vi "4463 and 4464 sync test.vi"() -> ()   [LabVIEW 2015]
uses:
  <vilib>/Analysis/1siggen.llb/Ramp Pattern by Samples.vi
  <vilib>/DAQmx/write.llb/DAQmx Write (Analog 1D DBL 1Chan NSamp).vi
  <vilib>/DAQmx/read.llb/DAQmx Read (Analog 1D DBL 1Chan NSamp).vi
  <vilib>/DAQmx/create/channels.llb/DAQmx Create Channel (AI-Voltage-Basic).vi
  <vilib>/DAQmx/configure/timing.llb/DAQmx Timing (Sample Clock).vi
  <vilib>/DAQmx/create/channels.llb/DAQmx Create Channel (AO-Voltage-Basic).vi
  <vilib>/DAQmx/configure/trigger.llb/DAQmx Start Trigger (Digital Edge).vi
  <vilib>/DAQmx/miscellaneous.llb/DAQmx Fill In Error Info.vi
  <resource>/objmgr/daqmx.rc
  <vilib>/Analysis/NI_AALBase.lvlib
panel:
  out "Graph":dbl[](graph)
  in  "stop":bool
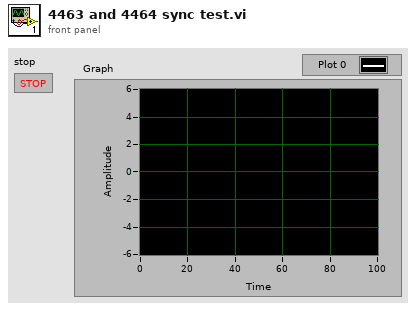
[diagram p1: front panel]
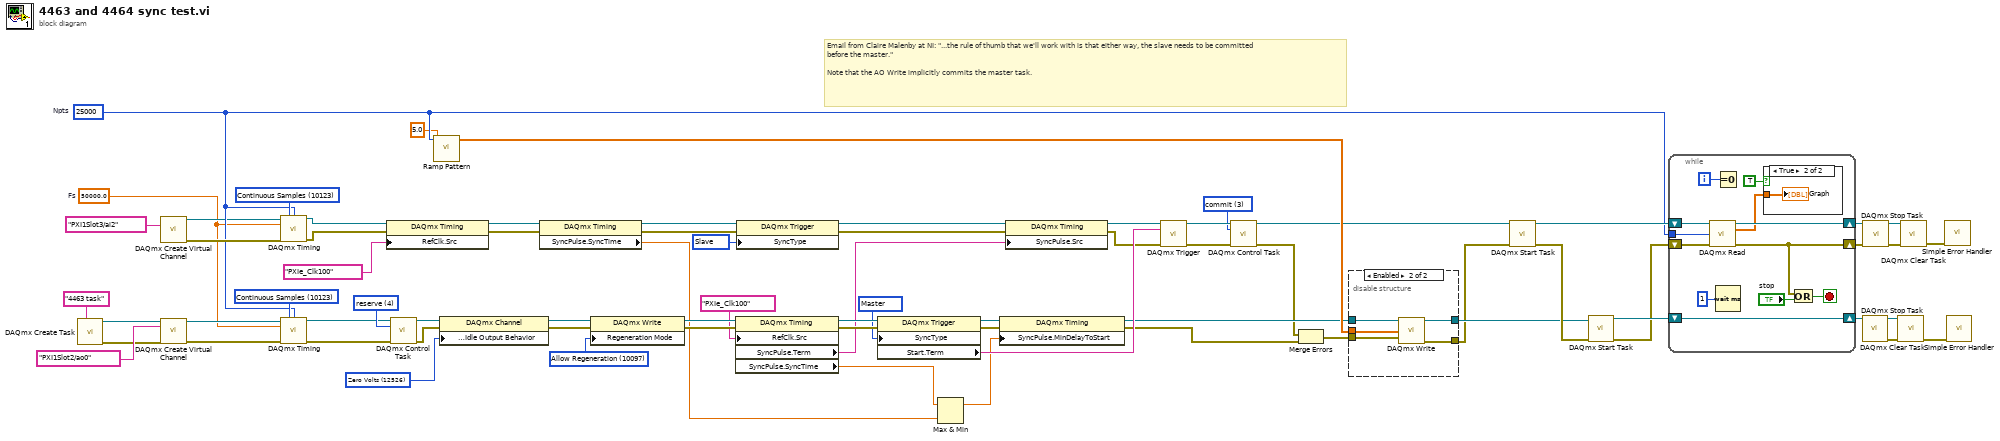
[diagram p0: block diagram]
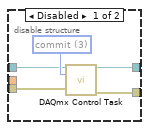
[diagram p2: hidden frame]
diagram:
  w1 = 3 items=["verify"=2, "reserve"=4, "commit"=3, "unreserve"=5, "abort"=6] ("action")
  w27 = 4 items=["verify"=2, "reserve"=4, "commit"=3, "unreserve"=5, "abort"=6] ("action")
  w33 = 12526 items=["Zero Volts"=12526, "High-Impedance"=12527, "Maintain Existing Value"=12528] ("AO.IdleOutputBehavior")
  w46 = 15889 items=["None"=10230, "Master"=15888, "Slave"=15889] ("SyncType")
  w47 = 15888 items=["None"=10230, "Master"=15888, "Slave"=15889] ("SyncType")
  w28 = 50000.0  # Fs
  w66 = 10123 items=["Finite Samples"=10178, "Continuous Samples"=10123, "Hardware Timed Single Point"=12522] ("sample mode")
  w69 = 10097 items=["Allow Regeneration"=10097, "Do Not Allow Regeneration"=10158] ("RegenMode")
  w37 = 25000  # Npts
  w71 = 10123 items=["Finite Samples"=10178, "Continuous Samples"=10123, "Hardware Timed Single Point"=12522] ("sample mode")
  # "Email from Claire Malenby at NI: \"...the rule of thumb that we'll work with is that either way, the slave needs to be committed before the master.\"\n\nNote that the AO Write implicitly commits the master task."
  n1 = call <vilib>:"DAQmx Create Task.vi"("new task name"="4463 task") -> ("task out"=w43:refnum<k21>, "error out"=w45:errorcluster)  [unwired: 13 in]
  n2 = call-poly <vilib>:"DAQmx Create Virtual Channel.vi"("physical channels"=tag "PXI1Slot3/ai2") -> ("task out"=w34:refnum<k21>, "error out"=w72:errorcluster)  [unwired: 13 in]
  n3 = call-poly <vilib>:"DAQmx Create Virtual Channel.vi"("task in"=w43, "physical channels"=tag "PXI1Slot2/ao0", "error in"=w45) -> ("task out"=w70:refnum<k21>, "error out"=w68:errorcluster)  [unwired: 11 in]
  n4 = call-poly <vilib>:"DAQmx Timing.vi"("task/channels in"=w34, "sample mode"=w71, "samples per channel"=w37, "rate"=w28, "error in"=w72) -> ("task out"=w51:refnum<k21>, "error out"=w50:errorcluster)  [unwired: 9 in]
  n5 = call-poly <vilib>:"DAQmx Timing.vi"("task/channels in"=w70, "sample mode"=w66, "samples per channel"=w37, "rate"=w28, "error in"=w68) -> ("task out"=w26:refnum<k21>, "error out"=w25:errorcluster)  [unwired: 9 in]
  n6 = property class="DAQmx Timing"(reference=w51, error in=w50, "RefClk.Src"=tag "PXIe_Clk100") -> (reference out=w31:refnum<k21>, error out=w42:errorcluster)
  n7 = call <vilib>:"DAQmx Control Task.vi"("task/channels in"=w26, "action"=w27, "error in"=w25) -> ("task out"=w24:refnum<k21>, "error out"=w23:errorcluster)  [unwired: 11 in]
  n8 = call-poly <vilib>:"Ramp Pattern.vi"("end"=5.0, "samples"=w37) -> ("Ramp Pattern"=w9:dbl[])  [unwired: 8 in, 1 out]
  n9 = property class="DAQmx Channel"(reference=w24, error in=w23, "Analog Output:General Properties:Output Configuration:Idle Output Behavior"=w33) -> (reference out=w30:refnum<k21>, error out=w29:errorcluster)
  n10 = property class="DAQmx Timing"(reference=w31, error in=w42) -> (reference out=w40:refnum<k21>, error out=w41:errorcluster, "SyncPulse.SyncTime"=w39:dbl)
  n11 = property class="DAQmx Write"(reference=w30, error in=w29, "Regeneration Mode"=w69) -> (reference out=w65:refnum<k21>, error out=w64:errorcluster)
  n12 = property class="DAQmx Timing"(reference=w65, error in=w64, "RefClk.Src"=tag "PXIe_Clk100") -> (reference out=w49:refnum<k21>, error out=w48:errorcluster, "SyncPulse.Term"=w15:tag, "SyncPulse.SyncTime"=w38:dbl)
  n13 = property class="DAQmx Trigger"(reference=w40, error in=w41, "SyncType"=w46) -> (reference out=w17:refnum<k21>, error out=w16:errorcluster)
  n14 = property class="DAQmx Trigger"(reference=w49, error in=w48, "SyncType"=w47) -> (reference out=w20:refnum<k21>, error out=w19:errorcluster, "Start.Term"=w18:tag)
  n15 = Max & Min(x=w38, y=w39) -> (max(x,y)=w12:dbl)  [unwired: 1 out]
  n16 = property class="DAQmx Timing"(reference=w20, error in=w19, "SyncPulse.MinDelayToStart"=w12) -> (reference out=w8:refnum<k21>, error out=w7:errorcluster)
  n17 = property class="DAQmx Timing"(reference=w17, error in=w16, "SyncPulse.Src"=w15) -> (reference out=w14:refnum<k21>, error out=w13:errorcluster)
  n18 = call-poly <vilib>:"DAQmx Trigger.vi"("task/channels in"=w14, "source"=w18, "error in"=w13) -> ("task out"=w5:refnum<k21>, "error out"=w6:errorcluster)  [unwired: 11 in]
  n19 = call <vilib>:"DAQmx Control Task.vi"("task/channels in"=w5, "action"=w1, "error in"=w6) -> ("task out"=w3:refnum<k21>, "error out"=w4:errorcluster)  [unwired: 11 in]
  n20 = Merge Errors(w4, w7) -> (w11:errorcluster)
  n21 = disable-structure shown="Enabled" {
    disable-tunnel: w11 -> [w76 w79]
    disable-tunnel: w8 -> [w75 w81]
    disable-tunnel: [w74 w80] -> w10
    disable-tunnel: [w73 w78] -> w2
    disable-tunnel: w9 -> [_ w82]
    frame Disabled {
      w77 = 3 items=["verify"=2, "reserve"=4, "commit"=3, "unreserve"=5, "abort"=6] ("action")
      n22 = call <vilib>:"DAQmx Control Task.vi"("task/channels in"=w75, "action"=w77, "error in"=w76) -> ("task out"=w74:refnum<k21>, "error out"=w73:errorcluster)  [unwired: 11 in]
    }
    frame Enabled {
      n23 = call-poly <vilib>:"DAQmx Write.vi"("task/channels in"=w81, "data"=w82, "error in"=w79) -> ("task out"=w80:refnum<k21>, "error out"=w78:errorcluster)  [unwired: 10 in, 1 out]
    }
  }
  n24 = call <vilib>:"DAQmx Start Task.vi"("task/channels in"=w3, "error in"=w2) -> ("task out"=w63:refnum<k21>, "error out"=w22:errorcluster)  [unwired: 12 in]
  n25 = call <vilib>:"DAQmx Start Task.vi"("task/channels in"=w10, "error in"=w22) -> ("task out"=w62:refnum<k21>, "error out"=w21:errorcluster)  [unwired: 12 in]
  n26 = while {
    tunnel: w37 -> [w88]
    shift-right: [w85] -> w60
    shift-left: w21 -> [w90]
    shift-right: [w92] -> w59
    shift-left: w62 -> [w92]
    shift-right: [w89] -> w61
    shift-left: w63 -> [w91]
    i -> [w84]
    stop <- w86 stop-if-true
    n27 = call-poly <vilib>:"DAQmx Read.vi"("task/channels in"=w91, "number of samples per channel"=w88, "error in"=w90) -> ("task out"=w89:refnum<k21>, "data"=w87:dbl[], "error out"=w85:errorcluster)  [unwired: 10 in]
    n28 = Equal To 0?(x=w84) -> ()  [unwired: 1 out]
    n29 = Wait (ms)(milliseconds to wait=u32 1) -> ()  [unwired: 1 out]
    n30 = case shown="True" TRUE {
      tunnel: w87 -> [_ w95]
      frame False {
      }
      frame True {
        "Graph" <- w95
      }
    }
    n31 = Or(x=w85, y="stop") -> (x .or. y?=w86:bool)
  }
  n32 = call <vilib>:"DAQmx Stop Task.vi"("task/channels in"=w59) -> ("task out"=w56:refnum<k21>, "error out"=w55:errorcluster)  [unwired: 13 in]
  n33 = call <vilib>:"DAQmx Stop Task.vi"("task/channels in"=w61, "error in"=w60) -> ("task out"=w58:refnum<k21>, "error out"=w57:errorcluster)  [unwired: 12 in]
  n34 = call <vilib>:"DAQmx Clear Task.vi"("task in"=w56, "error in"=w55) -> ("error out"=w52:errorcluster)  [unwired: 13 in]
  n35 = call <vilib>:"DAQmx Clear Task.vi"("task in"=w58, "error in"=w57) -> ("error out"=w32:errorcluster)  [unwired: 13 in]
  n36 = call <vilib>:"Simple Error Handler.vi"("error in (no error)"=w32) -> ()  [unwired: 4 in, 5 out]
  n37 = call <vilib>:"Simple Error Handler.vi"("error in (no error)"=w52) -> ()  [unwired: 4 in, 5 out]
